vi "Measure DC Current.vi"(8 "error in (no error)":errorcluster, 10 "measurementservice_SMUConfigResponse_Data":T1, 11 "SMUSession":refnum<k15>) -> (0 "error out":errorcluster, 1 "Compliance/Limit Reached":bool, 2 "Current Measurement":dbl, 3 "Voltage Measurement":dbl)   [LabVIEW 2019, in "ctet_smu User Library.lvlib"]
doc: "Demonstrates how to use the DC Current Output Function to force an output current. This example initializes a session, configures the Output Function, Sense, Autorange, Current Level and Voltage Limit, initiates generation, waits for a specified delay, and measures the voltage and current output. This example uses Single Point source mode."
uses:
  ctet_smu User Library.lvlib
  Servers/ctet_smu/ctet_smu Class/RPC Messages/measurementservice_SMUConfigResponse/measurementservice_SMUConfigResponse_Data.ctl
  Servers/ctet_smu/ctet_smu Class/RPC Messages/measurementservice_ErrorOut/measurementservice_ErrorOut_Data.ctl
  <instrlib>/niDCPower/nidcpower.llb/niDCPower Wait For Event - Event.ctl
  Servers/ctet_smu/ctet_smu Class/ctet_smu.lvclass
panel:
  # "Overview: Demonstrates how to use the DC Current Output Function to force an output current.  \nThis example initializes a session, configures the Output Function, Sense, Autorange, Current Level \nand Voltage Limit, initiates generation, waits for a specified delay, and measures the voltage and \ncurrent output.  \nRequirements: NI-DCPower\nInstructions:\n1. Select the appropriate device in the Resource Name control.\n2. Configure the parameters of the DC Current signal you'd like to output.\n3. Run the VI."
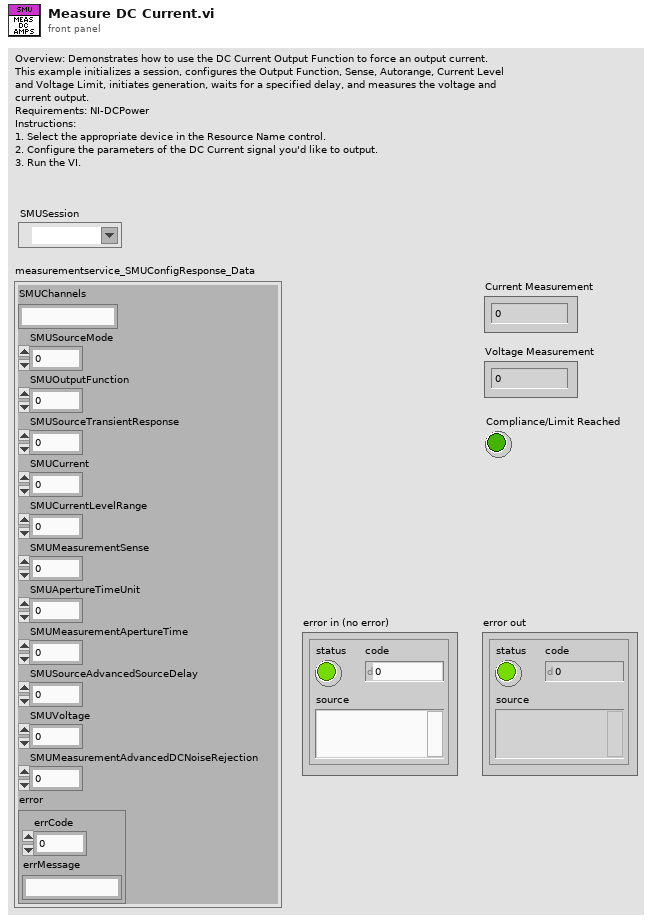
[diagram p1: front panel]
types:
  T1 = typedef "ctet_smu.lvlib/ctet_smu.lvclass/measurementservice_SMUConfigResponse_Data.ctl" = cluster{"SMUChannels":string, "SMUSourceMode":i64, "SMUOutputFunction":i64, "SMUSourceTransientResponse":i64, "SMUCurrent":dbl, "SMUCurrentLevelRange":dbl, "SMUMeasurementSense":i64, "SMUApertureTimeUnit":i64, "SMUMeasurementApertureTime":dbl, "SMUSourceAdvancedSourceDelay":dbl, "SMUVoltage":dbl, "SMUMeasurementAdvancedDCNoiseRejection":i64, "error":T2}
  T2 = typedef "ctet_smu.lvlib/ctet_smu.lvclass/measurementservice_ErrorOut_Data.ctl" = cluster{"errCode":i64, "errMessage":string}
  T3 = typedef "niDCPower Wait For Event - Event.ctl" = i32
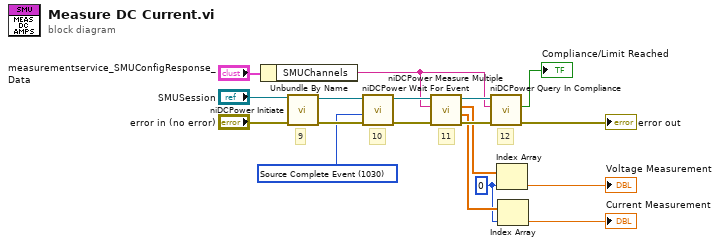
[diagram p0: block diagram]
diagram:
  w7 = T3 1030 items=["Source Complete Event"=1030, "Measure Complete Event"=1031, "Sequence Iteration Complete Event"=1032, "Sequence Engine Done Event"=1033] ("event")
  w12 = 0 ("index")
  # "11"
  # "10"
  # "12"
  # "9"
  n1 = Unbundle By Name("measurementservice_SMUConfigResponse_Data") -> ("SMUChannels"=w3:string)
  n2 = call <instrlib>:"niDCPower Initiate.vi"("error in (no error)"="error in (no error)", "instrument handle"="SMUSession") -> ("error out"=w9:errorcluster, "instrument handle out"=w11:refnum<k15>)  [unwired: 2 in, 6 out]
  n3 = call <instrlib>:"niDCPower Wait For Event.vi"("error in (no error)"=w9, "event"=w7, "instrument handle"=w11) -> ("error out"=w8:errorcluster, "instrument handle out"=w10:refnum<k15>)  [unwired: 1 in, 6 out]
  n4 = call <instrlib>:"niDCPower Measure Multiple.vi"("error in (no error)"=w8, "channel name"=w3, "instrument handle"=w10) -> ("error out"=w16:errorcluster, "current measurements"=w13:dbl[], "voltage measurements"=w14:dbl[], "instrument handle out"=w17:refnum<k15>)  [unwired: 5 out]
  n5 = call <instrlib>:"niDCPower Query In Compliance.vi"("error in (no error)"=w16, "channel name"=w3, "instrument handle"=w17) -> ("error out"=→"error out":errorcluster, "in compliance?"=→"Compliance/Limit Reached":bool)  [unwired: 7 out]
  n6 = Index Array(array=w14, index=w12) -> (element=→"Voltage Measurement":dbl)
  n7 = Index Array(array=w13, index=w12) -> (element=→"Current Measurement":dbl)
